vi "qLOG.vi"(0 "System no.":i32=1 min=1 max=4 step=1, 2 "Start Index":T3=-2147483648 min=1 max=4 step=1, 5 "error in":errorcluster) -> (14 "Array of LogInfo":T1 {"Error Code" min=1 max=4 step=1; "Index" min=1 max=4 step=1}, 19 "error out":errorcluster)   [LabVIEW 2026]
doc: "LOG? (Retrieve Error Log Lines)\n\nDescription\nQueries the contents of the log memory of the controller.\nDetails on the log memory:\nAfter switching on/rebooting the controller, all errors are logged in chronological order \nin a global log memory.\nThe log memory is volatile memory. Depending on the hardware, it can be \nimplemented as a ring buffer in which errors are stored according to the FIFO principle, \ni.e. the newest errors overwrite the oldest errors.\nAfter switching on/rebooting the controller, all errors are counted and marked in the \nlog memory with a consecutive index. Each error is also given a timestamp.\nA query with LOG? resets the bits for errors from the classes Critical, Info, and Warning in the \nstatus register of the system (p. 99). \nThe bit for errors of the Command class is reset in the status register of the system with the \nERR? command (p. 13). \n\nFormat\nLOG?[ <StartIndex>]\n\nArguments\n<StartIndex>\nLimitation of the query to certain errors\n= 1 queries all errors from the specified index onwards\n0 queries all errors stored in the log memory after LOG? was last sent on the currently used \ncommunication interface\n-n queries the errors last stored in the log memory, where n is the number of errors to query. If \nthe log memory holds less that the specified number of entries, all existing entries are \ndisplayed.\n\nResponse\nContents of the log memory, optionally limited to certain errors. \nOutput format:\nThe Error Information block consists of at least the following fields:\n- Index Consecutive number of the error\n- Timestamp Timestamp for the occurrence of the error in ns. UINT64\n- Error Code Bit-coded information containing the error class and error ID \n- Error Class Error class, also encoded in the error code. Note: Errors in classes Info, \nWarning, Command, Critical and Motion are displayed in a status register (p. 66). \n? Container Unit Alias (p. 94) for the container unit in which the error occurred\n? Function Unit Alias (p. 94) for the function unit in which the error occurred\nThe Error Information block also contains the following fields if the current user command level \nis >= Developer:\nLine Code Line in which the error occurred\nExample\n>>log?\n<<#Error Information: <Index> <Timestamp><Error Code>\n<Error Class> <Container Unit> <Function Unit>\n<<1 17375192000000 49155 CMD SYS_1 INTPR_1\n<<2 17628935000000 49217 CMD SYS_1 INTPR_1\n<<3 17780977000000 49155 CMD SYS_1 INTPR_1\n<<4 19842372000000 49154 CMD SYS_1 INTPR_1\n<<5 19854851000000 49155 CMD SYS_1 INTPR_1\n<<6 19906690000000 49169 CMD SYS_1 INTPR_1\n<<#END Error Information\n>>log? 3\n<<#Error Information: <Index> <Timestamp> <Error Code>\n<Error Class> <Container Unit><Function Unit>\n<<3 17780977000000 49155 CMD SYS_1 INTPR_1\n<<4 19842372000000 49154 CMD SYS_1 INTPR_1\n<<5 19854851000000 49155 CMD SYS_1 INTPR_1\n<<6 19906690000000 49169 CMD SYS_1 INTPR_1\n<<#END Error Information\n>>log? 6\n<<#Error Information: <Index> <Timestamp> <Error Code>\n<Error Class> <Container Unit><Function Unit>\n<<6 19906690000000 49169 CMD SYS_1 INTPR_1\n<<#END Error Information\n\nNotes\nAll entries of the log memory are output whose index is greater than or equal to the specified \nindex, even if the specified index is no longer contained in the memory (e.g. in the case of a ring \nbuffer).\nIn GCS 3.0, errors that occur during operation of the controller are recorded and output as \nfollows:\n- After switching on/rebooting the controller, all errors are logged globally and stored \ntemporarily. The contents of the log memory can be queried with the LOG? command\n(p. 21). \n- The ERR? command (p. 13) queries the error code that is currently stored in the GCS \ninterpreter of the communication interface used. Only errors of the Command class are \nstored in the GCS interpreters of the controller.\n- The status register of an axis (p. 97) shows whether an error of the Motion class is \npresent for the axis (i.e. a motion error). The status register of an axis can be queried \nwith the STV? command (p. 66). \n- The status register of the system (p. 99) shows whether there are errors from the \nclasses Command, Critical, Warning and Info. The status register of the system can be \nqueried with the STV? command (p. 66). \nUser software could, for example, use the bits of the status registers as trigger for querying the \nlog memory.\nFor further information, see \"Error Handling - GCS 3.0\" (p. 114). \n\nUser command level\nUSR"
uses:
  LOG_NoIndex.ctl
  Array of LogInfo.ctl
  LogInfo.ctl
panel:
  # "LOG? (Retrieve Error Log Lines)\n\nQueries the contents of the log memory of the controller.\nDetails on the log memory:\n- After switching on/rebooting the controller, all errors are logged in chronological order \nin a global log memory.\n- The log memory is volatile memory. Depending on the hardware, it can be \nimplemented as a ring buffer in which errors are stored according to the FIFO principle, \ni.e. the newest errors overwrite the oldest errors.\n- After switching on/rebooting the controller, all errors are counted and marked in the \nlog memory with a consecutive index. Each error is also given a timestamp.\nA query with LOG? resets the bits for errors from the classes Critical, Info, and Warning in the \nstatus register of the system (p. 99). \nThe bit for errors of the Command class is reset in the status register of the system with the \nERR? command (p. 13)."
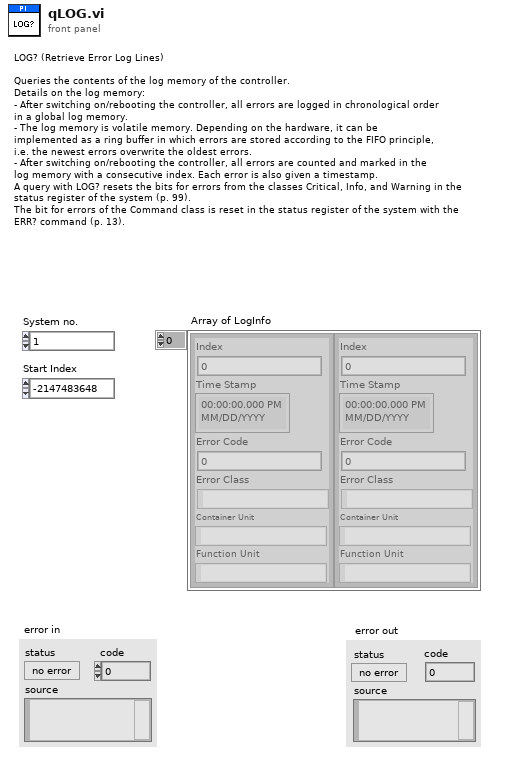
[diagram p1: front panel]
types:
  T1 = typedef "Array of LogInfo.ctl" = T2[]
  T2 = typedef "LogInfo.ctl" = cluster{"Index":i32, "Time Stamp":timestamp, "Error Code":i32, "Error Class":string, "Container Unit":string, "Function Unit":string}
  T3 = typedef "LOG_NoIndex.ctl" = i32
  T4 = typedef "Syntax.ctl" = enum16{"GCS 1.0", "GCS 2.0", "GCS 3.0"}
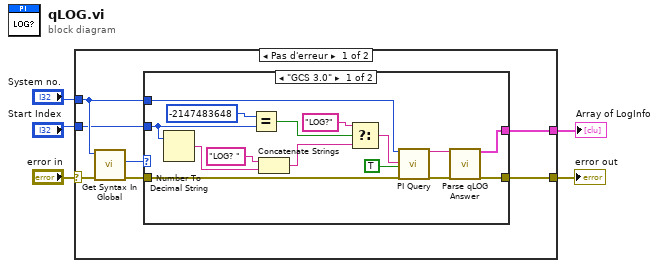
[diagram p0: block diagram]
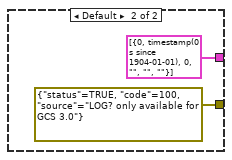
[diagram p2: hidden frame]
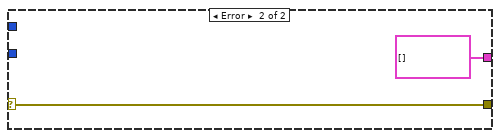
[diagram p3: hidden frame]
diagram:
  n1 = case shown="Pas d'erreur" "error in" {
    selector: "error in" -> [w11 w31]
    tunnel: [w12 w31] -> w5
    tunnel: "System no." -> [w8 _]
    tunnel: [w6 T2[] []] -> w1
    tunnel: "Start Index" -> [w7 _]
    frame No Error {
      n2 = call "Get Syntax In Global.vi"("error in"=w11, "System no."=w8) -> ("error out"=w10:errorcluster, "Syntax"=w9:T4)  [unwired: 8 in]
      n3 = case shown="\"GCS 3.0\"" w9 {
        tunnel: [w24 errorcluster {"status"=TRUE, "code"=100, "source"="LOG? only available for GCS 3.0"} ("error out")] -> w12
        tunnel: w8 -> [w23 _]
        tunnel: w10 -> [w22 _]
        tunnel: w7 -> [w16 _]
        tunnel: [w25 T2[] [{"Index"=0, "Time Stamp"=timestamp(0 s since 1904-01-01), "Error Code"=0, "Error Class"="", "Container Unit"="", "Function Unit"=""}]] -> w6
        frame "GCS 3.0" {
          n4 = Number To Decimal String(number=w16) -> (decimal integer string=w26:string)  [unwired: 1 in]
          n5 = Equal?(x=T3 -2147483648, y=w16) -> (x = y?=w15:bool)
          n6 = Concatenate Strings("LOG? ", w26) -> (w13:string)
          n7 = Select(t="LOG?", s=w15, f=w13) -> (s? t:f=w18:string)
          n8 = call "PI Query.vi"("System no."=w23, "String to send"=w18, "Attach termination char.?"=TRUE, "error in"=w22) -> ("String read"=w20:string, "error out"=w21:errorcluster)  [unwired: 12 in, 2 out]
          n9 = call "Parse qLOG Answer.vi"("Answer to Parse"=w20, "error in"=w21) -> ("Array of LogInfo"=w25:T2[], "error out"=w24:errorcluster)  [unwired: 16 in]
        }
        frame Default {
        }
      }
    }
    frame Error {
    }
  }
  "error out" <- w5
  "Array of LogInfo" <- w1
